vi "Logarithm10 of Number (U32).vi"(9 "Input Valid":bool=TRUE, 10 "Input Number (0.32)":fxp<+,32,0>) -> (1 "Output Valid":bool, 2 "Logarithm":fxp<+/-,34,12> format="%.26g", 4 "Exponent (-N)":i8, 6 "Mantissa (M)":fxp<+,32,0> format="%.0b")   [LabVIEW 2011]
doc: "This VI calculates the logarithm of a number in base 10\n\nAlgorithm:\n1) Convert the fixed point number into the form M*2^N (M is normalized FXP)\n\nMath: LOG(X)=LOG(M * 2^N)=LOG(M) + N*LOG(2) = LOG(M) + N* 0.301 \n\n2) To get Log (M) use a Look Up Table or BRAM\n\n3) Implement LOG(M) + n* 0.301 using DSP48E \n\n<b> Resources Used: </b>\n1) This code module uses a VI-Scoped BRAM of 512 elements\n\n<b> Latency = 11 Ticks </b>"
uses:
  <vilib>/rvi/DataTransferAndStorage/Container/Common/niFpgaContainerState.ctl
  <vilib>/rvi/DataTransferAndStorage/Container/Common/niFpgaDataTypeControl.ctl
  <vilib>/rvi/DataTransferAndStorage/Container/Common/niFpgaContainerImplementationControl.ctl
  <vilib>/rvi/DataTransferAndStorage/Container/Common/niFpgaContainerArbitrationOptionsControl.ctl
  <vilib>/rvi/DataTransferAndStorage/Container/Common/niFpgaTransferTypeControl.ctl
  <vilib>/rvi/DataTransferAndStorage/Container/Common/niFpgaContainerInitializationParameters.ctl
  <vilib>/rvi/Memory/Memory_Types/niFpgaMemoryInterfaceConfiguration.ctl
  <vilib>/rvi/FIFO/Fifo_Types/niFpgaFifoControlLogicControl.ctl
  <vilib>/rvi/DataTransferAndStorage/Container/Common/niFpgaContainerMetaDataKey.ctl
  <vilib>/rvi/DataTransferAndStorage/Container/Common/niFpgaContainerGetUniqueNameForEmu.vi
  <vilib>/rvi/DataTransferAndStorage/Container/Common/niFpgaContainerSetEmuInfo.vi
  <vilib>/rvi/eio/common/nirviEmuReportErrorAndStop.vi
  <vilib>/rvi/DataTransferAndStorage/Container/Common/niFpgaContainerExecOnDevCompGetState.vi
  <vilib>/rvi/Memory/Memory_Emulation/niFpgaMemoryEmulationValidateCache.vi
  <vilib>/rvi/Memory/Memory_Emulation/nirvimemoryEmulationManagerCache_InsertValue.vi
  <vilib>/Utility/error.llb/Clear Errors.vi
  <vilib>/rvi/Memory/Memory_Emulation/nirvimemoryEmulationManagerCache_GetValue.vi
  <vilib>/rvi/FXPMathLib/basic elements/FxpDiscreteDelay/XNode/nifxpmath_DiscreteDelay.xnode
  <vilib>/rvi/FXPMathLib/FxpInterpret/XNode/nifxpmath_Interpret.xnode
  <vilib>/rvi/LocalResourceManager/LocalResourceManager.xnode
  <vilib>/rvi/DataTransferAndStorage/Container/XNode/niFpgaContainer.xnode
  <vilib>/rvi/Memory/Memory_Emulation/niFpgaMemoryEmulationRefIn.vi
panel:
  out "Truncated Address":u16
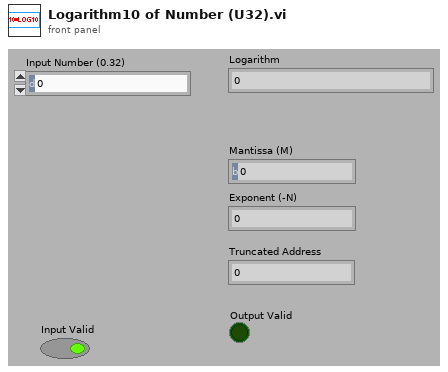
[diagram p1: front panel]
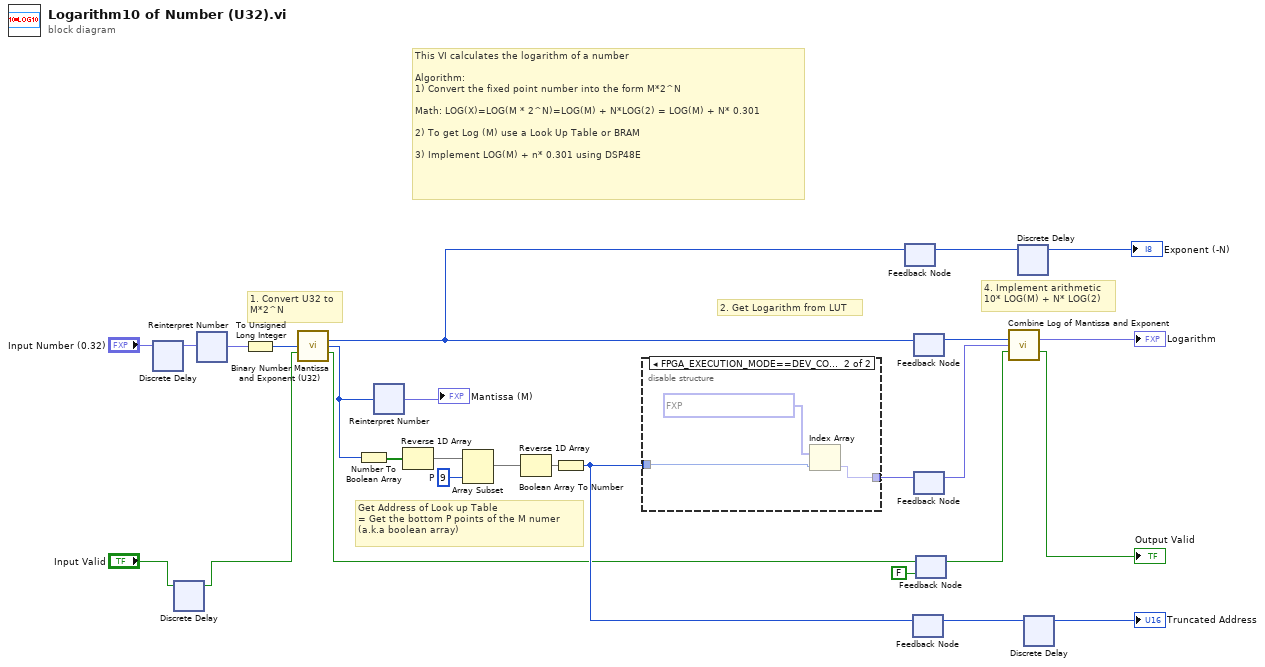
[diagram p0: block diagram]
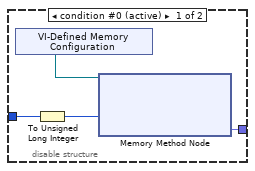
[diagram p2: hidden frame]
diagram:
  w25 = 9  # P
  # "4. Implement arithmetic\n10* LOG(M) + N* LOG(2)"
  # "2. Get Logarithm from LUT"
  # "1. Convert U32 to\nM*2^N"
  # "This VI calculates the logarithm of a number\n\nAlgorithm:\n1) Convert the fixed point number into the form M*2^N\n\nMath: LOG(X)=LOG(M * 2^N)=LOG(M) + N*LOG(2) = LOG(M) + N* 0.301 \n\n2) To get Log (M) use a Look Up Table or BRAM\n\n3) Implement LOG(M) + n* 0.301 using DSP48E"
  # "Get Address of Look up Table\n= Get the bottom P points of the M numer\n(a.k.a boolean array)"
  n1 = xnode "Discrete Delay"("D"="Input Number (0.32)") -> ("Q"=w8:fxp<+,32,0>)
  n2 = xnode "Discrete Delay"("D"="Input Valid") -> ("Q"=w1:bool)
  n3 = xnode "Reinterpret Number"("x"=w8) -> ("y"=w27:fxp<+,32,32>)
  n4 = To Unsigned Long Integer(number=w27) -> (unsigned 32bit integer=w26:u32)
  n5 = call <userlib>:"Binary Number Mantissa and Exponent (U32).vi"("Binary Number"=w26, "Input Valid"=w1) -> ("Exponent (-N)"=w20:i8, "Mantissa (M)"=w11:u32, "Output Valid"=w7:bool)  [unwired: 11 in]
  n6 = Number To Boolean Array(number=w11) -> (Boolean array=w24:bool[])
  n7 = xnode "Reinterpret Number"("x"=w11) -> ("y"=→"Mantissa (M)":fxp<+,32,0>)
  n8 = Reverse 1D Array(array=w24) -> (reversed array=w23:bool[])
  n9 = Array Subset(array=w23, length=w25) -> (w22:bool[])  [unwired: 1 in]
  n10 = Reverse 1D Array(array=w22) -> (reversed array=w21:bool[])
  n11 = Boolean Array To Number(Boolean array=w21) -> (number=w18:u16)
  n12 = disable-structure shown="FPGA_EXECUTION_MODE==DEV_COMPUTER_SIM_IO, default" {
    disable-tunnel: w18 -> [w31 w58]
    disable-tunnel: [w28 w57] -> w17
    frame condition #0 (active) {
      n13 = xnode "VI-Defined Memory Configuration"() -> ("Memory Out"=w29:refnum<k21>)
      n14 = To Unsigned Long Integer(number=w31) -> (unsigned 32bit integer=w30:u32)
      n15 = xnode ("Memory Method Node")("Address"=w30, "Memory In"=w29) -> ("Data"=w28:fxp<+/-,18,8>)  [unwired: 1 out]
    }
    frame condition #1 {
      n16 = Index Array(array=fxp<+/-,18,8>[] [-128.0, -27.0927734375, -24.08203125, -22.3212890625, -21.072265625, -20.1025390625, -19.3115234375, -18.6416015625, -18.0615234375, -17.5498046875, -17.0927734375, -16.6787109375, -16.30078125, -15.953125, -15.6318359375, -15.33203125, -15.0517578125, -14.7880859375, -14.5400390625, -14.3046875, -14.08203125, -13.8701171875, -13.6689453125, -13.4755859375, -13.291015625, -13.11328125, -12.943359375, -12.779296875, -12.62109375, -12.46875, -12.3212890625, -12.1787109375, -12.041015625, -11.9072265625, -11.7783203125, -11.65234375, -11.529296875, -11.4111328125, -11.294921875, -11.181640625, -11.072265625, -10.96484375, -10.8603515625, -10.7578125, -10.658203125, -10.560546875, -10.46484375, -10.3720703125, -10.2802734375, -10.1904296875, -10.1025390625, -10.0166015625, -9.9326171875, -9.849609375, -9.7685546875, -9.689453125, -9.6103515625, -9.5341796875, -9.4580078125, -9.3837890625, -9.3115234375, -9.2392578125, -9.1689453125, -9.099609375, -9.03125, -8.9638671875, -8.8974609375, -8.83203125, -8.767578125, -8.7041015625, -8.6416015625, -8.580078125, -8.51953125, -8.458984375, -8.400390625, -8.341796875, -8.2841796875, -8.2275390625, -8.171875, -8.1162109375, -8.0615234375, -8.0078125, -7.9541015625, -7.90234375, -7.849609375, -7.798828125, -7.748046875, -7.697265625, -7.6474609375, -7.5986328125, -7.5498046875, -7.501953125, -7.455078125, -7.408203125, -7.361328125, -7.3154296875, -7.26953125, -7.224609375, -7.1806640625, -7.13671875, -7.0927734375, -7.0498046875, -7.0068359375, -6.9638671875, -6.9228515625, -6.880859375, -6.83984375, -6.798828125, -6.7587890625, -6.71875, -6.6787109375, -6.6396484375, -6.6005859375, -6.5615234375, -6.5234375, -6.4853515625, -6.4482421875, -6.4111328125, -6.3740234375, -6.3369140625, -6.30078125, -6.2646484375, -6.2294921875, -6.193359375, -6.158203125, -6.1240234375, -6.0888671875, -6.0546875, -6.0205078125, -5.986328125, -5.953125, -5.919921875, -5.88671875, -5.8544921875, -5.8212890625, -5.7890625, -5.7568359375, -5.7255859375, -5.6943359375, -5.662109375, -5.6318359375, -5.6005859375, -5.5693359375, -5.5390625, -5.5087890625, -5.4794921875, -5.44921875, -5.419921875, -5.3896484375, -5.3603515625, -5.33203125, -5.302734375, -5.2744140625, -5.24609375, -5.2177734375, -5.189453125, -5.1611328125, -5.1337890625, -5.1064453125, -5.0791015625, -5.0517578125, -5.0244140625, -4.9970703125, -4.970703125, -4.9443359375, -4.91796875, -4.8916015625, -4.865234375, -4.83984375, -4.8134765625, -4.7880859375, -4.7626953125, -4.7373046875, -4.7119140625, -4.6875, -4.662109375, -4.6376953125, -4.61328125, -4.5888671875, -4.564453125, -4.5400390625, -4.515625, -4.4921875, -4.4677734375, -4.4443359375, -4.4208984375, -4.3974609375, -4.3740234375, -4.3515625, -4.328125, -4.3046875, -4.2822265625, -4.259765625, -4.2373046875, -4.21484375, -4.1923828125, -4.169921875, -4.1484375, -4.1259765625, -4.1044921875, -4.08203125, -4.060546875, -4.0390625, -4.017578125, -3.99609375, -3.9755859375, -3.9541015625, -3.9326171875, -3.912109375, -3.8916015625, -3.8701171875, -3.849609375, -3.8291015625, -3.80859375, -3.7880859375, -3.7685546875, -3.748046875, -3.728515625, -3.7080078125, -3.6884765625, -3.6689453125, -3.6484375, -3.62890625, -3.609375, -3.58984375, -3.5712890625, -3.5517578125, -3.5322265625, -3.513671875, -3.494140625, -3.4755859375, -3.45703125, -3.4375, -3.4189453125, -3.400390625, -3.3818359375, -3.36328125, -3.345703125, -3.3271484375, -3.30859375, -3.291015625, -3.2724609375, -3.2548828125, -3.236328125, -3.21875, -3.201171875, -3.18359375, -3.166015625, -3.1484375, -3.130859375, -3.11328125, -3.095703125, -3.0791015625, -3.0615234375, -3.0439453125, -3.02734375, -3.0107421875, -2.9931640625, -2.9765625, -2.9599609375, -2.943359375, -2.9267578125, -2.91015625, -2.8935546875, -2.876953125, -2.8603515625, -2.84375, -2.8271484375, -2.8115234375, -2.794921875, -2.779296875, -2.7626953125, -2.7470703125, -2.7314453125, -2.71484375, -2.69921875, -2.68359375, -2.66796875, -2.65234375, -2.63671875, -2.62109375, -2.60546875, -2.58984375, -2.5751953125, -2.5595703125, -2.5439453125, -2.529296875, -2.513671875, -2.4990234375, -2.4833984375, -2.46875, -2.4541015625, -2.4384765625, -2.423828125, -2.4091796875, -2.39453125, -2.3798828125, -2.365234375, -2.3505859375, -2.3359375, -2.3212890625, -2.306640625, -2.29296875, -2.2783203125, -2.263671875, -2.25, -2.2353515625, -2.2216796875, -2.20703125, -2.193359375, -2.1787109375, -2.1650390625, -2.1513671875, -2.1376953125, -2.123046875, -2.109375, -2.095703125, -2.08203125, -2.068359375, -2.0546875, -2.041015625, -2.02734375, -2.013671875, -2.0009765625, -1.9873046875, -1.9736328125, -1.9609375, -1.947265625, -1.93359375, -1.9208984375, -1.9072265625, -1.89453125, -1.880859375, -1.8681640625, -1.85546875, -1.841796875, -1.8291015625, -1.81640625, -1.8037109375, -1.791015625, -1.7783203125, -1.765625, -1.751953125, -1.740234375, -1.7275390625, -1.71484375, -1.7021484375, -1.689453125, -1.6767578125, -1.6640625, -1.65234375, -1.6396484375, -1.626953125, -1.615234375, -1.6025390625, -1.5908203125, -1.578125, -1.56640625, -1.5537109375, -1.5419921875, -1.529296875, -1.517578125, -1.505859375, -1.4931640625, -1.4814453125, -1.4697265625, -1.4580078125, -1.4462890625, -1.4345703125, -1.4228515625, -1.4111328125, -1.3994140625, -1.3876953125, -1.3759765625, -1.3642578125, -1.3525390625, -1.3408203125, -1.3291015625, -1.3173828125, -1.306640625, -1.294921875, -1.283203125, -1.2724609375, -1.2607421875, -1.2490234375, -1.23828125, -1.2265625, -1.2158203125, -1.2041015625, -1.193359375, -1.181640625, -1.1708984375, -1.16015625, -1.1484375, -1.1376953125, -1.126953125, -1.1162109375, -1.1044921875, -1.09375, -1.0830078125, -1.072265625, -1.0615234375, -1.05078125, -1.0400390625, -1.029296875, -1.0185546875, -1.0078125, -0.9970703125, -0.986328125, -0.9755859375, -0.96484375, -0.9541015625, -0.943359375, -0.93359375, -0.9228515625, -0.912109375, -0.9013671875, -0.8916015625, -0.880859375, -0.8701171875, -0.8603515625, -0.849609375, -0.83984375, -0.8291015625, -0.8193359375, -0.80859375, -0.798828125, -0.7880859375, -0.7783203125, -0.7685546875, -0.7578125, -0.748046875, -0.73828125, -0.7275390625, -0.7177734375, -0.7080078125, -0.6982421875, -0.6875, -0.677734375, -0.66796875, -0.658203125, -0.6484375, -0.638671875, -0.62890625, -0.619140625, -0.609375, -0.599609375, -0.58984375, -0.580078125, -0.5703125, -0.560546875, -0.55078125, -0.541015625, -0.53125, -0.5224609375, -0.5126953125, -0.5029296875, -0.4931640625, -0.484375, -0.474609375, -0.46484375, -0.4560546875, -0.4462890625, -0.4365234375, -0.427734375, -0.41796875, -0.4091796875, -0.3994140625, -0.390625, -0.380859375, -0.3720703125, -0.3623046875, -0.353515625, -0.34375, -0.3349609375, -0.326171875, -0.31640625, -0.3076171875, -0.298828125, -0.2890625, -0.2802734375, -0.271484375, -0.2626953125, -0.2529296875, -0.244140625, -0.2353515625, -0.2265625, -0.2177734375, -0.208984375, -0.19921875, -0.1904296875, -0.181640625, -0.1728515625, -0.1640625, -0.1552734375, -0.146484375, -0.1376953125, -0.12890625, -0.1201171875, -0.111328125, -0.1025390625, -0.0947265625, -0.0859375, -0.0771484375, -0.068359375, -0.0595703125, -0.05078125, -0.04296875, -0.0341796875, -0.025390625, -0.0166015625, -0.0087890625] ("Init Data Out"), index=w58) -> (element=w57:fxp<+/-,18,8>)
    }
  }
  n17 = feedback-in #1(w20) -> ()
  n18 = feedback #1() -> (w6:i8)  [unwired: 1 in]
  n19 = feedback-in #2(w18) -> ()
  n20 = feedback #2() -> (w5:u16)  [unwired: 1 in]
  n21 = feedback-in #3(w20) -> ()
  n22 = feedback #3() -> (w14:i8)  [unwired: 1 in]
  n23 = feedback-in #4(w17) -> ()
  n24 = feedback #4() -> (w15:fxp<+/-,18,8>)  [unwired: 1 in]
  n25 = feedback #5(FALSE ("Input Valid")) -> (w13:bool)
  n26 = feedback-in #5(w7) -> ()
  n27 = call <userlib>:"Combine Log of Mantissa and Exponent.vi"("Exponent of 2"=w14, "10Log (Mantissa)"=w15, "Input Valid"=w13) -> ("Logarithm"=→"Logarithm":fxp<+/-,34,12>, "Output Valid"=→"Output Valid":bool)  [unwired: 11 in]
  n28 = xnode "Discrete Delay"("D"=w6) -> ("Q"=→"Exponent (-N)":i8)
  n29 = xnode "Discrete Delay"("D"=w5) -> ("Q"=→"Truncated Address":u16)
